vi "DDS9959 Set FR2.vi"(4 "error in (no error)":errorcluster, 6 "Channel Function Register":T1, 7 "VISA resource name":refnum<visa-resource-name>) -> (0 "error out":errorcluster, 3 "VISA resource name out":refnum<visa-resource-name>)   [LabVIEW 2012]
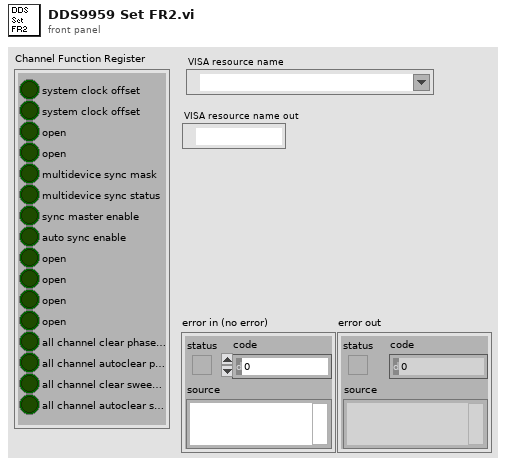
[diagram p1: front panel]
types:
  T1 = cluster{"system clock offset":bool, "system clock offset":bool, "open":bool, "open":bool, "multidevice sync mask":bool, "multidevice sync status":bool, "sync master enable":bool, "auto sync enable":bool, "open":bool, "open":bool, "open":bool, "open":bool, "all channel clear phase accumulator":bool, "all channel autoclear phase accumulator":bool, "all channel clear sweep accumulator":bool, "all channel autoclear sweep accumulator":bool}
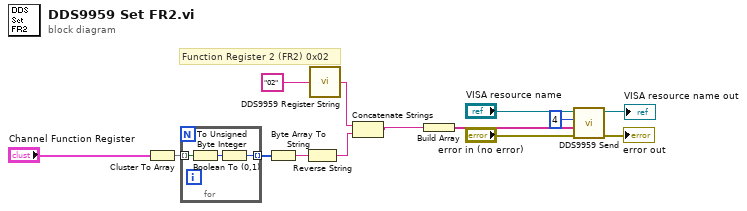
[diagram p0: block diagram]
diagram:
  # "Function Register 2 (FR2) 0x02"
  n1 = Cluster To Array(cluster="Channel Function Register") -> (array=w2:bool[])
  n2 = for {
    tunnel: w2 -> [w15] mode=indexing
    tunnel: [w16] -> w5 mode=indexing
    n3 = Boolean To (0,1)(Boolean=w15) -> (0, 1=w17:i16)
    n4 = To Unsigned Byte Integer(number=w17) -> (unsigned 8bit integer=w16:u8)
  }
  n5 = Byte Array To String(unsigned byte array=w5) -> (string=w4:string)
  n6 = Reverse String(1:w4) -> (0:w3:string)
  n7 = call "DDS9959 Register String.vi"("register"="02") -> ("output"=w9:string)
  n8 = Concatenate Strings(w9, w3) -> (w8:string)
  n9 = Build Array(w8) -> (w14:string[])
  n10 = call "DDS9959 Send.vi"("error in (no error)"="error in (no error)", "Output Array"=w14, "USB Out Endpoint"=i16 4, "VISA resource name"="VISA resource name") -> ("error out"=→"error out":errorcluster, "VISA resource name"=→"VISA resource name out":refnum<visa-resource-name>)  [unwired: 6 in]
